vi "RemoveZeros.vi"(11 "spectrum in":dbl[](array[numeric])) -> (3 "Spectrum":dbl[](array[numeric]))   [LabVIEW 2018]
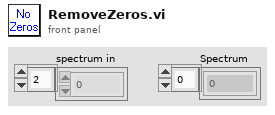
[diagram p1: front panel]
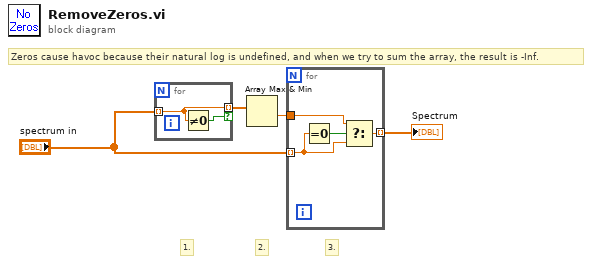
[diagram p0: block diagram]
diagram:
  # "3."
  # "2."
  # "1."
  # "Zeros cause havoc because their natural log is undefined, and when we try to sum the array, the result is -Inf."
  n1 = for {
    tunnel: "spectrum in" -> [w6] mode=indexing
    tunnel: [w6] -> w1 mode=indexing if=w5
    n2 = Not Equal To 0?(x=w6) -> (x != 0?=w5:bool)
  }
  n3 = Array Max & Min(array=w1) -> (min value=w4:dbl)  [unwired: 3 out]
  n4 = for {
    tunnel: "spectrum in" -> [w9] mode=indexing
    tunnel: w4 -> [w8]
    tunnel: [w7] -> w3 mode=indexing
    n5 = Equal To 0?(x=w9) -> (x = 0?=w10:bool)
    n6 = Select(t=w8, s=w10, f=w9) -> (s? t:f=w7:dbl)
  }
  "Spectrum" <- w3
